vi "GetImage.vi"(8 "error in (no error)":errorcluster, 11 "reference in":refnum<class "Camera_IMAQdx.lvclass">) -> (0 "error out":errorcluster, 2 "Image":T1, 3 "reference out":refnum<class "Camera_IMAQdx.lvclass">)   [LabVIEW 2017, in "Camera_IMAQdx.lvclass"]
doc: "Gets image reference"
uses:
  Camera_IMAQdx.lvclass
  <vilib>/vision/Image Controls.llb/IMAQ Image.ctl
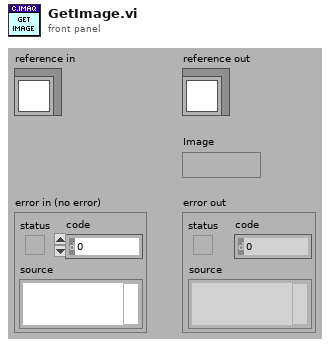
[diagram p1: front panel]
types:
  T1 = typedef "IMAQ Image.ctl" = refnum<image>
  T2 = typedef "Camera_IMAQdx.lvclass/ObjectAttributes.ctl" = cluster{"Configuration":T3, "Session":T4, "Connected":bool, "Image":T1, "Grab Frame Number":u32}
  T3 = typedef "Camera_IMAQdx.lvclass/Configuration--Cluster.ctl" = cluster{"Camera Interface Name":string, "Number of Buffers":u32, "Image Name":string}
  T4 = typedef "IMAQdx.ctl" = refnum<k21>
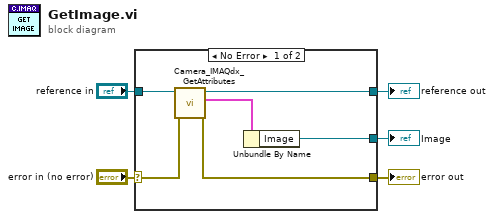
[diagram p0: block diagram]
diagram:
  n1 = case shown="No Error" "error in (no error)" {
    selector: "error in (no error)" -> [w11 w13]
    tunnel: [w9 w13] -> w4
    tunnel: [w7 w12] -> w2
    tunnel: "reference in" -> [w8 w12]
    tunnel: [w6 _] -> w1
    frame No Error {
      n2 = call "Camera_IMAQdx_GetAttributes.vi"("error in (no error)"=w11, "reference in"=w8) -> ("error out"=w9:errorcluster, "Data"=w10:T2, "reference out"=w7:refnum<class "Camera_IMAQdx.lvclass">)  [unwired: 6 in, 1 out]
      n3 = Unbundle By Name(w10) -> ("Image"=w6:T1)
    }
    frame Error {
    }
  }
  "error out" <- w4
  "reference out" <- w2
  "Image" <- w1
